vi "setVcselPulsePeriod.vi"(7 "vcselPeriodType":T9(ring), 8 "error in":errorcluster, 9 "period_pclks":u8, 10 "Slave Address (7-bit)":u8, 11 "I2C Ref In":T1) -> (0 "error out":errorcluster, 2 "status":bool, 3 "I2C Ref Out":T1)   [LabVIEW 2018]
uses:
  <vilib>/myRIO/Instrument Drivers/Onboard IO/I2C/typedefs/I2C Reference.ctl
  <vilib>/myRIO/Common/Instrument Driver Framework/Utilities/typedefs/myRIO Generic Hardware Reference.ctl
  <vilib>/myRIO/Common/Instrument Driver Framework/Utilities/typedefs/Hardware Version Enum.ctl
  <vilib>/myRIO/Common/Instrument Driver Framework/Utilities/typedefs/myRIO v1.0 Reference.ctl
  <vilib>/myRIO/Common/Instrument Driver Framework/Utilities/typedefs/Generic FPGA Reference.ctl
  <vilib>/myRIO/Common/Instrument Driver Framework/myRIO v1.0/I2C/typedefs/I2C Channels Enum.ctl
  <vilib>/myRIO/Instrument Drivers/Onboard IO/I2C/typedefs/I2C Configuration.ctl
  <vilib>/myRIO/Instrument Drivers/Onboard IO/I2C/typedefs/I2C Transfer Rate.ctl
  <vilib>/Utility/error.llb/Error Cluster From Error Code.vi
  <vilib>/myRIO/Common/Instrument Driver Framework/myRIO v1.0/I2C/vis/myRIO v1.0 Write I2C.vi
  <vilib>/myRIO/Instrument Drivers/Onboard IO/I2C/I2C.lvlib
panel:
  # "NOTE: NOT YET DEBUG!!!!!!!!!!!!!!!!!!!!!!!!!!!!11!!"
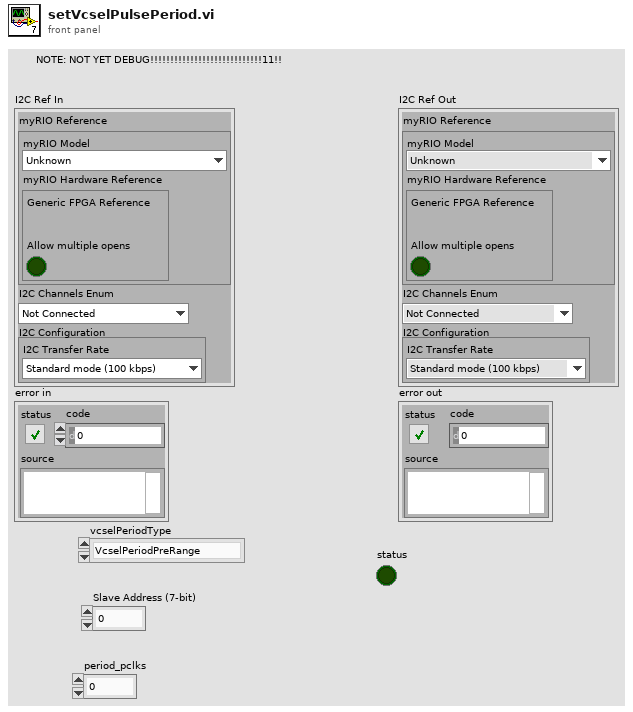
[diagram p1: front panel]
types:
  T1 = typedef "I2C.lvlib/I2C Reference.ctl" = cluster{"myRIO Reference":T2, "I2C Channels Enum":T6, "I2C Configuration":T7}
  T2 = typedef "myRIO Generic Hardware Reference.ctl" = cluster{"myRIO Model":T3, "myRIO Hardware Reference":T4}
  T3 = typedef "Hardware Version Enum.ctl" = enum16{"Unknown", "myRIO-1900", "myRIO-1950", "roboRIO", "NI ELVIS RIO CM", "ELVIS III"}
  T4 = typedef "myRIO v1.0 Reference.ctl" = cluster{"Generic FPGA Reference":T5, "Allow multiple opens":bool}
  T5 = typedef "Generic FPGA Reference.ctl" = refnum<k20>
  T6 = typedef "I2C Channels Enum.ctl" = enum16{"Not Connected", "A/I2C", "B/I2C", "I2C/I2C"}
  T7 = typedef "I2C.lvlib/I2C Configuration.ctl" = cluster{"I2C Transfer Rate":T8}
  T8 = typedef "I2C.lvlib/I2C Transfer Rate.ctl" = enum16{"Standard mode (100 kbps)", "Fast mode (400 kbps)"}
  T9 = enum8{"VcselPeriodPreRange", "VcselPeriodFinalRange"}
  T10 = cluster{"tcc":bool, "dss":bool, "msrc":bool, "pre_range":bool, "final_range":bool}
  T11 = cluster{"pre_range_vcsel_period_pclks":u16, "final_range_vcsel_period_pclks":u16, "msrc_dss_tcc_mclks":u16, "pre_range_mclks":u16, "final_range_mclks":u16, "msrc_dss_tcc_us":u32, "pre_range_us":u32, "final_range_us":u32}
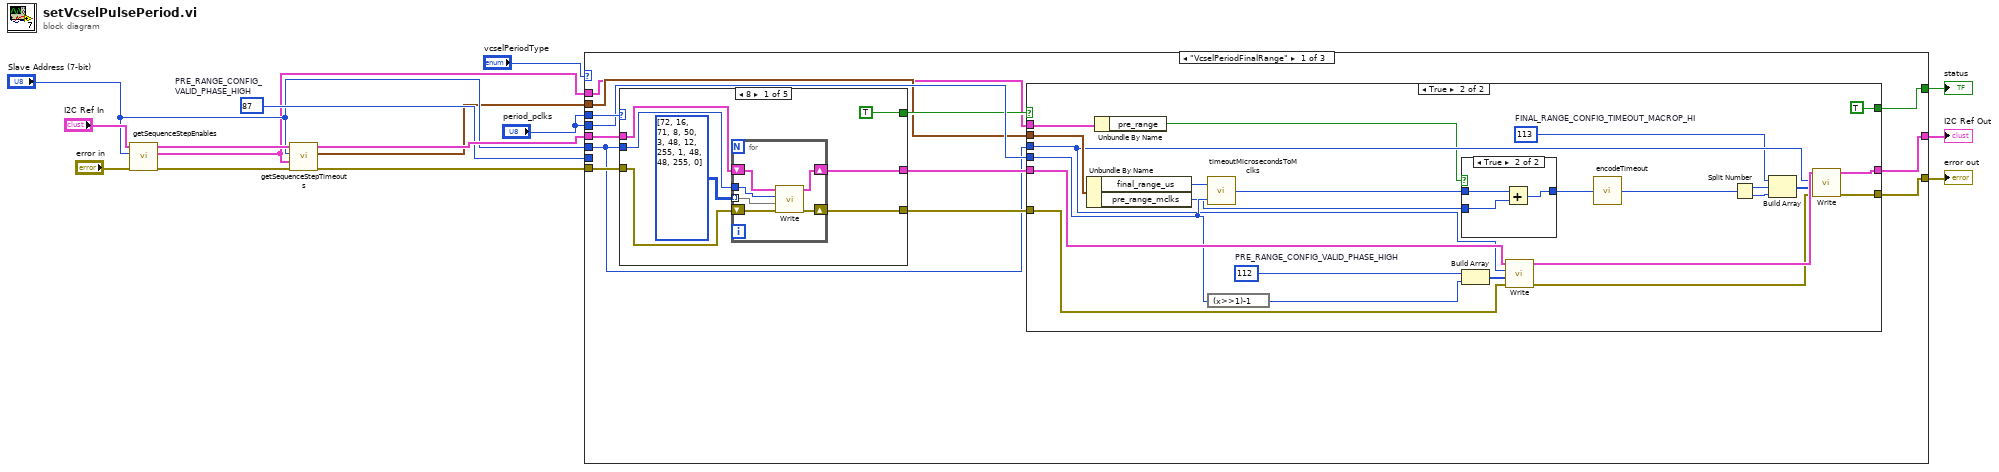
[diagram p0: block diagram]
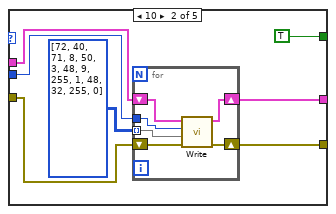
[diagram p4: hidden frame]
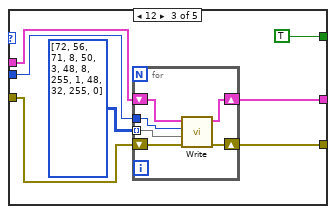
[diagram p5: hidden frame]
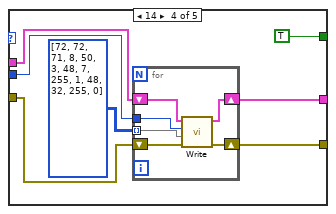
[diagram p6: hidden frame]
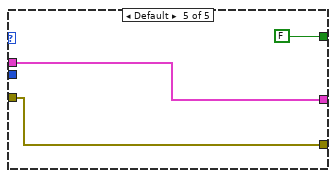
[diagram p7: hidden frame]
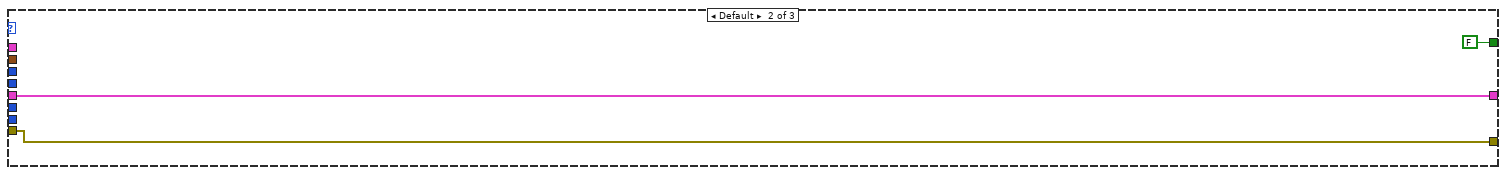
[diagram p8: hidden frame]
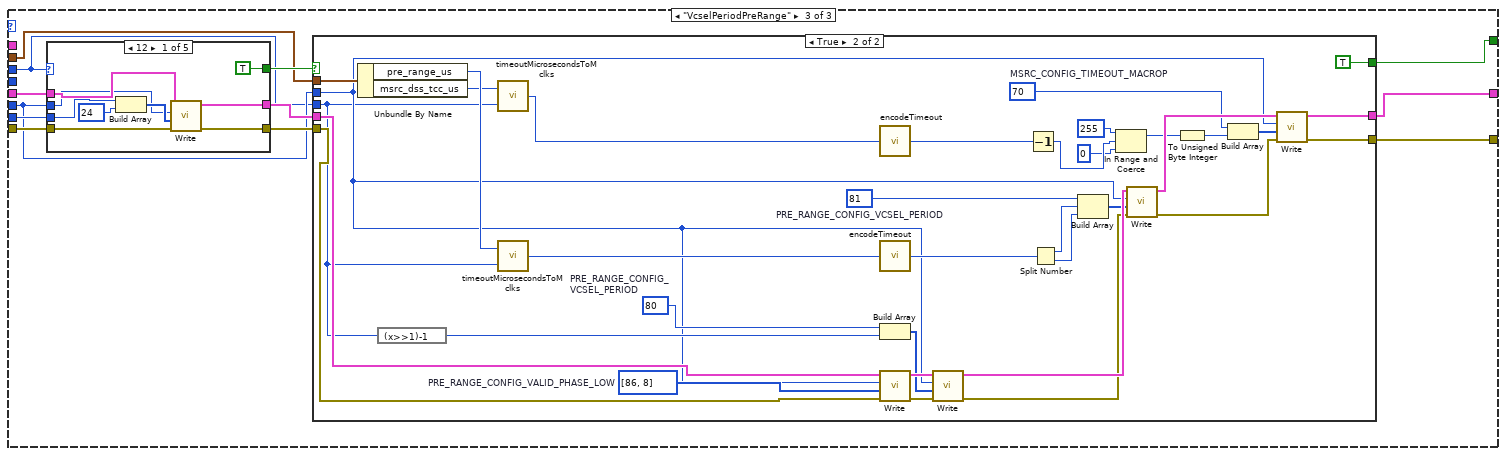
[diagram p9: hidden frame]
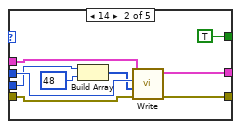
[diagram p11: hidden frame]
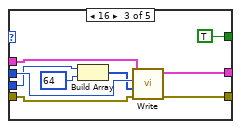
[diagram p12: hidden frame]
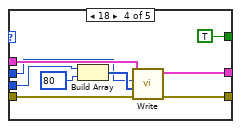
[diagram p13: hidden frame]
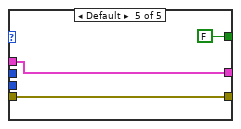
[diagram p14: hidden frame]
diagram:
  w9 = u8 87  # PRE_RANGE_CONFIG_VALID_PHASE_HIGH
  n1 = call "getSequenceStepEnables.vi"("error in"="error in", "Slave Address (7-bit)"="Slave Address (7-bit)", "I2C Ref In"="I2C Ref In") -> ("error out"=w12:errorcluster, "enables"=w1:T10, "I2C Ref Out"=w14:T1)  [unwired: 6 in]
  n2 = call "getSequenceStepTimeouts.vi"("error in"=w12, "enables"=w1, "Slave Address (7-bit)"="Slave Address (7-bit)", "I2C Ref In"=w14) -> ("error out"=w10:errorcluster, "timeouts"=w7:T11, "I2C Ref Out"=w11:T1)  [unwired: 4 in]
  n3 = case shown="\"VcselPeriodFinalRange\"" "vcselPeriodType" {
    tunnel: "period_pclks" -> [w28 _ w118]
    tunnel: w11 -> [w27 w116 w129]
    tunnel: w10 -> [w26 w115 w128]
    tunnel: w9 -> [_ _ w127]
    tunnel: "Slave Address (7-bit)" -> [w22 _ w123]
    tunnel: w7 -> [w19 _ w122]
    tunnel: [w20 FALSE w121] -> w6
    tunnel: [w18 w116 w120] -> w5
    tunnel: [w17 w115 w119] -> w4
    tunnel: "period_pclks" -> [w25 _ _]
    tunnel: w1 -> [w16 _ _]
    frame "VcselPeriodFinalRange" {
      n4 = case shown="8" w28 {
        tunnel: [TRUE TRUE TRUE TRUE FALSE] -> w21
        tunnel: w22 -> [w64 w75 w88 w101 _]
        tunnel: w27 -> [w63 w77 w90 w103 w113]
        tunnel: w26 -> [w62 w76 w89 w102 w112]
        tunnel: [w61 w74 w87 w100 w113] -> w24
        tunnel: [w60 w73 w86 w99 w112] -> w23
        frame 8 {
          n5 = for {
            tunnel: u8[][] [[72, 16], [71, 8], [50, 3], [48, 12], [255, 1], [48, 48], [255, 0]] -> [w71] mode=indexing
            tunnel: w64 -> [w72]
            shift-right: [w67] -> w60
            shift-left: w62 -> [w69]
            shift-right: [w68] -> w61
            shift-left: w63 -> [w70]
            n6 = call <vilib>:"Write.vi"("error in (no error)"=w69, "Bytes to Write"=w71, "Slave Address (7-bit)"=w72, "I2C Ref In"=w70) -> ("error out"=w67:errorcluster, "I2C Ref Out"=w68:T1)  [unwired: 6 in]
          }
        }
        frame 10 {
          n7 = for {
            tunnel: u8[][] [[72, 40], [71, 8], [50, 3], [48, 9], [255, 1], [48, 32], [255, 0]] -> [w84] mode=indexing
            tunnel: w75 -> [w85]
            shift-right: [w80] -> w73
            shift-left: w76 -> [w82]
            shift-right: [w81] -> w74
            shift-left: w77 -> [w83]
            n8 = call <vilib>:"Write.vi"("error in (no error)"=w82, "Bytes to Write"=w84, "Slave Address (7-bit)"=w85, "I2C Ref In"=w83) -> ("error out"=w80:errorcluster, "I2C Ref Out"=w81:T1)  [unwired: 6 in]
          }
        }
        frame 12 {
          n9 = for {
            tunnel: u8[][] [[72, 56], [71, 8], [50, 3], [48, 8], [255, 1], [48, 32], [255, 0]] -> [w97] mode=indexing
            tunnel: w88 -> [w98]
            shift-right: [w93] -> w86
            shift-left: w89 -> [w95]
            shift-right: [w94] -> w87
            shift-left: w90 -> [w96]
            n10 = call <vilib>:"Write.vi"("error in (no error)"=w95, "Bytes to Write"=w97, "Slave Address (7-bit)"=w98, "I2C Ref In"=w96) -> ("error out"=w93:errorcluster, "I2C Ref Out"=w94:T1)  [unwired: 6 in]
          }
        }
        frame 14 {
          n11 = for {
            tunnel: u8[][] [[72, 72], [71, 8], [50, 3], [48, 7], [255, 1], [48, 32], [255, 0]] -> [w110] mode=indexing
            tunnel: w101 -> [w111]
            shift-right: [w106] -> w99
            shift-left: w102 -> [w108]
            shift-right: [w107] -> w100
            shift-left: w103 -> [w109]
            n12 = call <vilib>:"Write.vi"("error in (no error)"=w108, "Bytes to Write"=w110, "Slave Address (7-bit)"=w111, "I2C Ref In"=w109) -> ("error out"=w106:errorcluster, "I2C Ref Out"=w107:T1)  [unwired: 6 in]
          }
        }
        frame Default {
        }
      }
      n13 = case shown="True" w21 {
        selector: w21 -> [w31 _]
        tunnel: w25 -> [_ w49]
        tunnel: w24 -> [w30 w53]
        tunnel: w23 -> [w29 w52]
        tunnel: w22 -> [_ w44]
        tunnel: [w31 TRUE] -> w20
        tunnel: w19 -> [_ w50]
        tunnel: [w30 w35] -> w18
        tunnel: [w29 w34] -> w17
        tunnel: w16 -> [_ w33]
        frame False {
        }
        frame True {
          w43 = u8 113  # FINAL_RANGE_CONFIG_TIMEOUT_MACROP_HI
          w55 = u8 112  # PRE_RANGE_CONFIG_VALID_PHASE_HIGH
          n14 = Unbundle By Name(w50) -> ("final_range_us"=w48:u32, "pre_range_mclks"=w47:u16)
          n15 = Unbundle By Name(w33) -> ("pre_range"=w32:bool)
          n16 = call "timeoutMicrosecondsToMclks.vi"("vcsel_period_pclks"=w49, "timeout_period_us"=w48) -> ("timeout_period_mclks"=w42:u32)
          n17 = expression code="(x>>1)-1"(w49) -> (w54:u8)
          n18 = case shown="True" w32 {
            tunnel: w42 -> [w56 w58]
            tunnel: w47 -> [_ w59]
            tunnel: [w56 w57] -> w41
            frame False {
            }
            frame True {
              n19 = Add(x=w58, y=w59) -> (x+y=w57:u32)
            }
          }
          n20 = Build Array(w55, w54) -> (w51:u8[])
          n21 = call <vilib>:"Write.vi"("error in (no error)"=w52, "Bytes to Write"=w51, "Slave Address (7-bit)"=w44, "I2C Ref In"=w53) -> ("error out"=w45:errorcluster, "I2C Ref Out"=w46:T1)  [unwired: 6 in]
          n22 = call "encodeTimeout.vi"("timeout_mclks"=w41) -> ("reg_val"=w39:u16)
          n23 = Split Number(x=w39) -> (hi(x)=w38:u8, lo(x)=w37:u8)
          n24 = Build Array(w43, w38, w37) -> (w40:u8[])
          n25 = call <vilib>:"Write.vi"("error in (no error)"=w45, "Bytes to Write"=w40, "Slave Address (7-bit)"=w44, "I2C Ref In"=w46) -> ("error out"=w34:errorcluster, "I2C Ref Out"=w35:T1)  [unwired: 6 in]
        }
      }
    }
    frame Default {
    }
    frame "VcselPeriodPreRange" {
      n26 = case shown="12" w118 {
        tunnel: [TRUE TRUE TRUE TRUE FALSE] -> w126
        tunnel: w129 -> [w173 w180 w193 w201 w205]
        tunnel: w128 -> [w172 w181 w192 w198 w204]
        tunnel: w123 -> [w168 w179 w191 w195 _]
        tunnel: w127 -> [w174 w177 w189 w196 _]
        tunnel: [w170 w183 w187 w200 w205] -> w125
        tunnel: [w171 w182 w186 w199 w204] -> w124
        frame 12 {
          n27 = Build Array(w174, u8 24) -> (w169:u8[])
          n28 = call <vilib>:"Write.vi"("error in (no error)"=w172, "Bytes to Write"=w169, "Slave Address (7-bit)"=w168, "I2C Ref In"=w173) -> ("error out"=w171:errorcluster, "I2C Ref Out"=w170:T1)  [unwired: 6 in]
        }
        frame 14 {
          n29 = Build Array(w177, u8 48) -> (w178:u8[])
          n30 = call <vilib>:"Write.vi"("error in (no error)"=w181, "Bytes to Write"=w178, "Slave Address (7-bit)"=w179, "I2C Ref In"=w180) -> ("error out"=w182:errorcluster, "I2C Ref Out"=w183:T1)  [unwired: 6 in]
        }
        frame 16 {
          n31 = Build Array(w189, u8 64) -> (w190:u8[])
          n32 = call <vilib>:"Write.vi"("error in (no error)"=w192, "Bytes to Write"=w190, "Slave Address (7-bit)"=w191, "I2C Ref In"=w193) -> ("error out"=w186:errorcluster, "I2C Ref Out"=w187:T1)  [unwired: 6 in]
        }
        frame 18 {
          n33 = Build Array(w196, u8 80) -> (w197:u8[])
          n34 = call <vilib>:"Write.vi"("error in (no error)"=w198, "Bytes to Write"=w197, "Slave Address (7-bit)"=w195, "I2C Ref In"=w201) -> ("error out"=w199:errorcluster, "I2C Ref Out"=w200:T1)  [unwired: 6 in]
        }
        frame Default {
        }
      }
      n35 = case shown="True" w126 {
        selector: w126 -> [w132 _]
        tunnel: [w132 TRUE] -> w121
        tunnel: w125 -> [w131 w167]
        tunnel: w124 -> [w130 w166]
        tunnel: w123 -> [_ w137]
        tunnel: w122 -> [_ w159]
        tunnel: [w131 w135] -> w120
        tunnel: [w130 w134] -> w119
        tunnel: w118 -> [_ w133]
        frame False {
        }
        frame True {
          w141 = u8 70  # MSRC_CONFIG_TIMEOUT_MACROP
          w153 = u8 81  # PRE_RANGE_CONFIG_VCSEL_PERIOD
          w161 = u8 80  # PRE_RANGE_CONFIG_VCSEL_PERIOD
          w165 = u8[] [86, 8]  # PRE_RANGE_CONFIG_VALID_PHASE_LOW
          n36 = Unbundle By Name(w159) -> ("pre_range_us"=w158:u32, "msrc_dss_tcc_us"=w148:u32)
          n37 = expression code="(x>>1)-1"(w133) -> (w160:u8)
          n38 = call "timeoutMicrosecondsToMclks.vi"("vcsel_period_pclks"=w133, "timeout_period_us"=w148) -> ("timeout_period_mclks"=w149:u32)
          n39 = call "timeoutMicrosecondsToMclks.vi"("vcsel_period_pclks"=w133, "timeout_period_us"=w158) -> ("timeout_period_mclks"=w157:u32)
          n40 = call "encodeTimeout.vi"("timeout_mclks"=w149) -> ("reg_val"=w147:u16)
          n41 = call "encodeTimeout.vi"("timeout_mclks"=w157) -> ("reg_val"=w156:u16)
          n42 = Build Array(w161, w160) -> (w162:u8[])
          n43 = call <vilib>:"Write.vi"("error in (no error)"=w166, "Bytes to Write"=w165, "Slave Address (7-bit)"=w137, "I2C Ref In"=w167) -> ("error out"=w163:errorcluster, "I2C Ref Out"=w164:T1)  [unwired: 6 in]
          n44 = call <vilib>:"Write.vi"("error in (no error)"=w163, "Bytes to Write"=w162, "Slave Address (7-bit)"=w137, "I2C Ref In"=w164) -> ("error out"=w151:errorcluster, "I2C Ref Out"=w152:T1)  [unwired: 6 in]
          n45 = Decrement(x=w147) -> (x-1=w145:u16)
          n46 = Split Number(x=w156) -> (hi(x)=w154:u8, lo(x)=w155:u8)
          n47 = Build Array(w153, w154, w155) -> (w150:u8[])
          n48 = In Range and Coerce(upper limit=u16 255, x=w145, lower limit=u16 0) -> (coerced(x)=w140:u16)  [unwired: 1 out]
          n49 = call <vilib>:"Write.vi"("error in (no error)"=w151, "Bytes to Write"=w150, "Slave Address (7-bit)"=w137, "I2C Ref In"=w152) -> ("error out"=w142:errorcluster, "I2C Ref Out"=w143:T1)  [unwired: 6 in]
          n50 = To Unsigned Byte Integer(number=w140) -> (unsigned 8bit integer=w138:u8)
          n51 = Build Array(w141, w138) -> (w139:u8[])
          n52 = call <vilib>:"Write.vi"("error in (no error)"=w142, "Bytes to Write"=w139, "Slave Address (7-bit)"=w137, "I2C Ref In"=w143) -> ("error out"=w134:errorcluster, "I2C Ref Out"=w135:T1)  [unwired: 6 in]
        }
      }
    }
  }
  "I2C Ref Out" <- w5
  "error out" <- w4
  "status" <- w6
